vi "LvMPDC_CMD_Database_update.vi"(6 "timeout_ms":i32=25000, 8 "error in (no error)":errorcluster, 9 "ReadBytes":i32=1024, 10 "pathext":string, 11 "Connect ID":refnum<k5>) -> (0 "error out":errorcluster, 3 "Connect ID out":refnum<k5>)   [LabVIEW 2012]
panel:
  # "LvMPDC:: CMD update (Databse)"
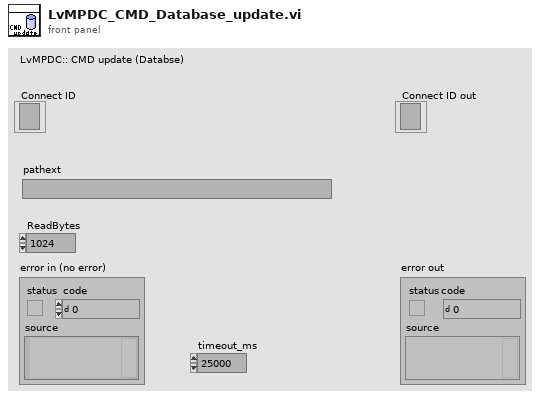
[diagram p1: front panel]
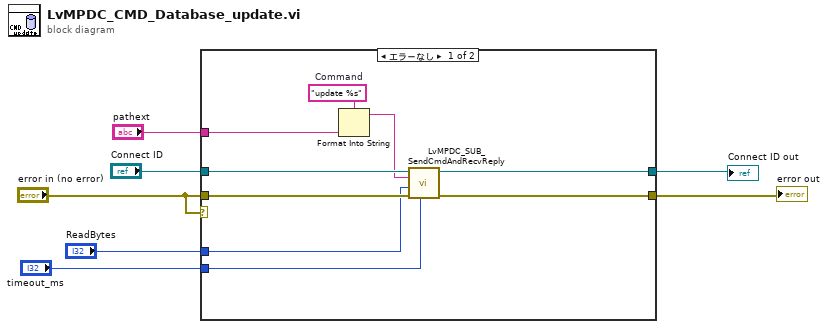
[diagram p0: block diagram]
diagram:
  n1 = case shown="エラーなし" "error in (no error)" {
    tunnel: "Connect ID" -> [w14 w18]
    tunnel: "error in (no error)" -> [w16 w17]
    tunnel: [w13 w18] -> w6
    tunnel: [w15 w17] -> w5
    tunnel: "timeout_ms" -> [w11 _]
    tunnel: "ReadBytes" -> [w12 _]
    tunnel: "pathext" -> [w10 _]
    frame No Error {
      w9 = "update %s"  # Command
      n2 = Format Into String(format string=w9, w10) -> (resulting string=w8:string)  [unwired: 2 in, 1 out]
      n3 = call "LvMPDC_SUB_SendCmdAndRecvReply.vi"("timeout_ms"=w11, "error in (no error)"=w16, "ReadBytes"=w12, "Command"=w8, "Connect ID"=w14) -> ("error out"=w15:errorcluster, "Connect ID out"=w13:refnum<k5>)  [unwired: 4 in, 1 out]
    }
    frame Error {
    }
  }
  "Connect ID out" <- w6
  "error out" <- w5
